vi "Test enum to string.vi"() -> ()   [LabVIEW 2019, in "Instrument-VIM.lvlib"]
uses:
  Instrument-VIM.lvlib
  b95be834-838a-46c0-a103-ccf79b46d759.vi
  97061c39-901d-49d9-9773-b5b8f94cdda8.vi
  a588928e-b79e-47fd-8b2f-27266a521fd2.vi
  a46d76b3-4efe-4f1f-b7b6-6a97a4340745.vi
  <vilib>/Utility/Data Type/Get Type Information.vi
  <vilib>/Utility/Data Type/Get Numeric Information.vi
  <userlib>/_OpenG.lib/lvdata/lvdata.llb/Unwrap VVariant__ogtk.vi
panel:
  out "string to variant to string":string[](array[string])
  out "enum to variant to string":string[](array[string])
  out "string to string":string[](array[string])
  out "enum to string":string[](array[string])
  out "string to variant to string":string
  out "enum to variant to string":string
  out "enum to string":string
  out "string to string":string
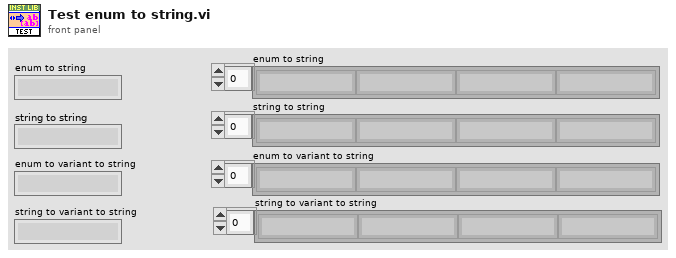
[diagram p1: front panel]
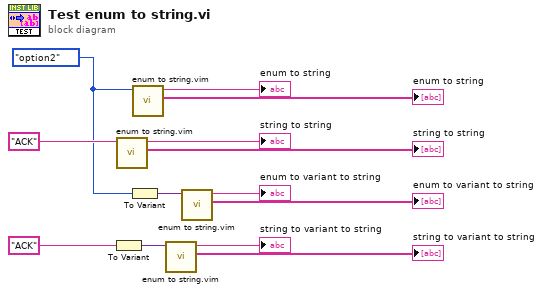
[diagram p0: block diagram]
diagram:
  w1 = enum16{"option1", "option2"}."option2"
  n1 = To Variant(anything="ACK") -> (Variant=w6:variant)
  n2 = call "enum to string.vim"("enum in"="ACK") -> ("strings out"=→"string to string":string[], "string out"=→"string to string":string)  [unwired: 9 in]
  n3 = To Variant(anything=w1) -> (Variant=w7:variant)
  n4 = call "enum to string.vim"("enum in"=w1) -> ("strings out"=→"enum to string":string[], "string out"=→"enum to string":string)  [unwired: 9 in]
  n5 = call "enum to string.vim"("enum in"=w6) -> ("strings out"=→"string to variant to string":string[], "string out"=→"string to variant to string":string)  [unwired: 9 in]
  n6 = call "enum to string.vim"("enum in"=w7) -> ("strings out"=→"enum to variant to string":string[], "string out"=→"enum to variant to string":string)  [unwired: 9 in]
